vi "Add Scale.vi"(8 "error in (no error)":errorcluster, 11 "Scaling configuration in":refnum<class "Scaling configuration.lvclass">) -> (0 "error out":errorcluster, 2 "new index":i32, 3 "Scaling configuration out":refnum<class "Scaling configuration.lvclass">)   [LabVIEW 2013, in "Scaling configuration.lvclass"]
uses:
  Scaling configuration.lvclass
  <vilib>/NI/Tag Bus Module Framework/channel/TBM channel.lvclass
  controls/scale data types.ctl
  Scaling configuration.lvclass/Scaling configuration.ctl
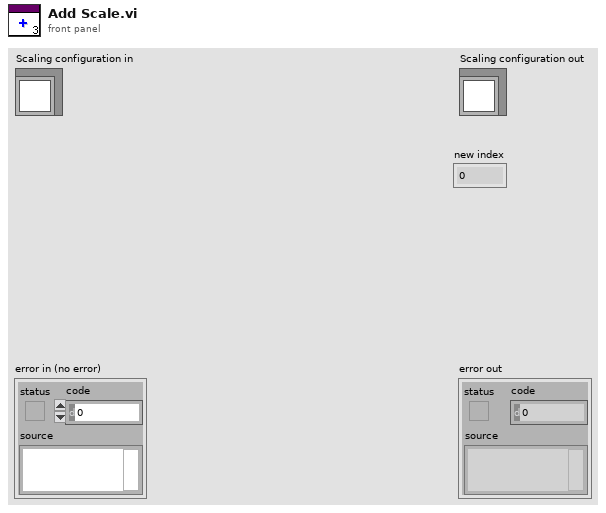
[diagram p1: front panel]
types:
  T1 = typedef "Scaling configuration.lvclass/scale data types.ctl" = enum16{"Double", "Single", "I64", "I32", "I16", "I8", "U64", "U32", "U16", "U8", "Boolean"}
  T2 = cluster{"mappings":cluster{"input channel":refnum<class "TBM channel.lvclass">, "output channel":refnum<class "TBM channel.lvclass">, "input data type":T1, "output data type":T1}[], "name":string}
  T3 = cluster{"mappings":cluster{"input channel":refnum<class "TBM channel.lvclass">, "output channel":refnum<class "TBM channel.lvclass">, "input data type":T1, "output data type":T1}[], "name":string}[]
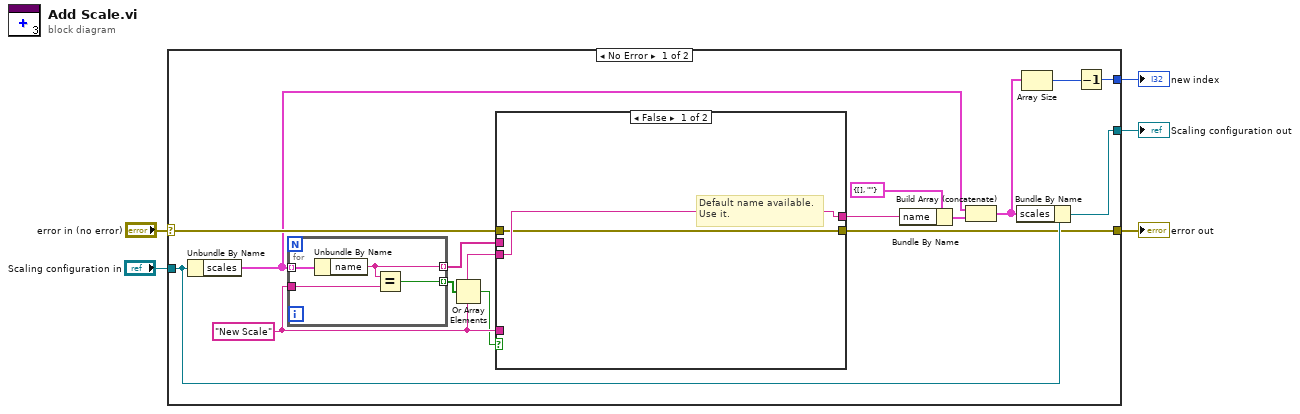
[diagram p0: block diagram]
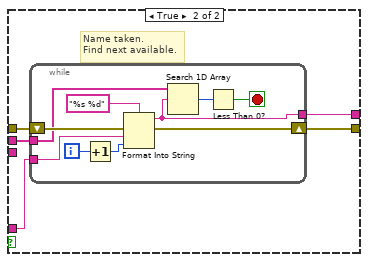
[diagram p2: hidden frame]
diagram:
  n1 = case shown="No Error" "error in (no error)" {
    selector: "error in (no error)" -> [w20 w43]
    tunnel: [w17 w43] -> w4
    tunnel: [w18 w42] -> w2
    tunnel: "Scaling configuration in" -> [w19 w42]
    tunnel: [w15 _] -> w1
    frame No Error {
      w14 = "New Scale" ("element")
      n2 = Unbundle By Name(w19) -> ("scales"=w12:T3)
      n3 = for {
        tunnel: w12 -> [w24] mode=indexing
        tunnel: w14 -> [w23]
        tunnel: [w22] -> w7 mode=indexing
        tunnel: [w21] -> w13 mode=indexing
        n4 = Unbundle By Name(w24) -> ("name"=w21:string)
        n5 = Equal?(x=w21, y=w23) -> (x = y?=w22:bool)
      }
      n6 = Or Array Elements(Boolean array=w7) -> (logical OR=w6:bool)
      n7 = case shown="False" w6 {
        tunnel: [w26 w31] -> w10
        tunnel: [w25 w30] -> w17
        tunnel: w13 -> [_ w29]
        tunnel: w14 -> [_ w28]
        tunnel: w14 -> [w26 _]
        tunnel: w20 -> [w25 w27]
        frame False {
          # "Default name available.\nUse it."
        }
        frame True {
          # "Name taken.\nFind next available."
          n8 = while {
            tunnel: [w36] -> w31
            shift-right: [w34] -> w30
            shift-left: w27 -> [w35]
            tunnel: w29 -> [w33]
            tunnel: w28 -> [w32]
            i -> [w40]
            stop <- w37 stop-if-true
            n9 = Increment(x=w40) -> (x+1=w39:i32)
            n10 = Format Into String(format string="%s %d", error in=w35, w32, w39) -> (resulting string=w36:string, error out=w34:errorcluster)  [unwired: 1 in]
            n11 = Search 1D Array(1D array=w33, element=w36) -> (index of element=w38:i32)  [unwired: 1 in]
            n12 = Less Than 0?(x=w38) -> (x < 0?=w37:bool)
          }
        }
      }
      n13 = Bundle By Name(cluster=T2 {"mappings"=[], "name"=""} ("Cluster"), "name"=w10) -> (w9:T2)
      n14 = Build Array (concatenate)(w12, w9) -> (w8:T3)
      n15 = Bundle By Name(cluster=w19, "scales"=w8) -> (w18:refnum<class "Scaling configuration.lvclass">)
      n16 = Array Size(array=w8) -> (size(s)=w16:i32)
      n17 = Decrement(x=w16) -> (x-1=w15:i32)
    }
    frame Error {
    }
  }
  "error out" <- w4
  "Scaling configuration out" <- w2
  "new index" <- w1
